vi "Set Mouse Position.vi"(1 "Y":i32, 2 "X":i32) -> ()   [LabVIEW 2015]
uses:
  USER32.DLL
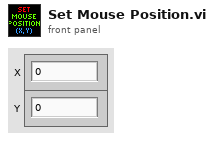
[diagram p1: front panel]
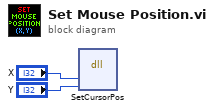
[diagram p0: block diagram]
diagram:
  n1 = dll-call lib="user32.dll" fn="SetCursorPos"("X"="X", "Y"="Y") -> ()  [unwired: 6 in, 2 out]
